vi "Test-Sideways Motors.vi"() -> ()   [LabVIEW 2014, in "Comp Driver.lvlib"]
uses:
  Comp Robot/Comp Drive/Comp Driver.lvlib
  Robot Actor Framework/Trace/Trace Controller Class/Config.ctl
  Comp Robot/Comp Motors with Encoders/Comp Motors with Encoders Class/Motor Controller Config.ctl
  Robot/Motor with Encoders/Motors with Encoders Class/Motors with Encoders Config.ctl
  Comp Robot/Comp Motors with Encoders/Comp Motors with Encoders Class/Encoder Config.ctl
  Comp Robot/Comp Trace Controller/Comp Trace Controller Class/Comp Trace Controller.lvclass
  Comp Robot/Comp Motors with Encoders/Comp Motors with Encoders Class/Comp Motors with Encoders.lvclass
  Comp Robot/Comp Pressure/Comp Pressure Class/Comp Pressure.lvclass
  <vilib>/Rock Robotics/WPI/DriverStation/WPI_DriverStationRobotMode2.ctl
  Robot/Motor with Encoders/Motors with Encoders Messages/Set Rate (Percent) Msg/Set Rate (Percent) Msg.lvclass/Set Rate (Percent) Msg.ctl
  <vilib>/ActorFramework/Message Enqueuer/Message Enqueuer.lvclass/Message Enqueuer.ctl
  <vilib>/ActorFramework/Message Enqueuer/Enqueue.vi
  <vilib>/ActorFramework/Message Priority Queue/Priority Enqueue.vi
  Robot/Motor with Encoders/Motors with Encoders Messages/Set Rate (Percent) Msg/Set Rate (Percent) Msg.lvclass
  <vilib>/ActorFramework/Stop Msg/Stop Msg.lvclass
  <vilib>/ActorFramework/Actor/Actor.lvclass
  Robot Actor Framework/Trace/Trace Controller Class/Trace Controller.lvclass
  Robot/Motor with Encoders/Motors with Encoders Class/Motors with Encoders.lvclass
panel:
  in  "Encoder Config":T1={"P"=1.0, "D"=0.0, "F"=0.01, "I"=0.01, "Reverse Feedback Sensor"=FALSE, "Encoder Codes Per Rev"=256}
  out "Enable Tele":bool caption="Enabled Teleop"
  in  "Stop Test Loop 1":bool=TRUE
  in  "Finish Test":bool=TRUE
  in  "Start Test":bool=TRUE
  in  "Rate (Percent)":dbl(slide)=-1.0 scale=-1.0..1.0
  in  "Motos with Encoder Config":T2={"Counts  Per Revolution"=256, "Invert Encoder Direction"=FALSE, "Diameter of Revolution"=6.0, "Max RPM"=1500.0, "Encoder Control"=TRUE}
  in  "Slave Motor Controller Configs":T3[](array[typedef])=[{"Device Number"=6, "Invert Motor"=FALSE}]
  in  "Master Motor Controller Config":T3={"Device Number"=11, "Invert Motor"=FALSE}
  in  "Trace Controller Config":T4={"Folder Pattern"="/media/sd%s1", "Starting Letter Position"=1, "Min Free Space (MB)"=50.0, "Max Folders to Check"=10, "Trace Level"=enum."Debug"} {"Min Free Space (MB)" format="%#_13g"}
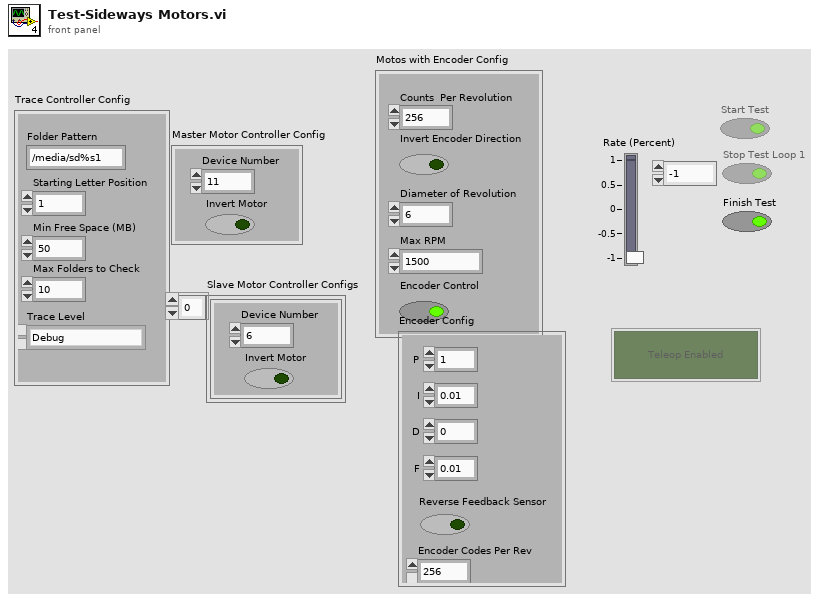
[diagram p1: front panel]
types:
  T1 = typedef "Comp Motors with Encoders.lvlib/Comp Motors with Encoders.lvclass/Encoder Config.ctl" = cluster{"P":dbl, "D":dbl, "F":dbl, "I":dbl, "Reverse Feedback Sensor":bool, "Encoder Codes Per Rev":u16}
  T2 = typedef "Motors with Encoders.lvlib/Motors with Encoders.lvclass/Motors with Encoders Config.ctl" = cluster{"Counts  Per Revolution":u32, "Invert Encoder Direction":bool, "Diameter of Revolution":dbl, "Max RPM":dbl, "Encoder Control":bool}
  T3 = typedef "Comp Motors with Encoders.lvlib/Comp Motors with Encoders.lvclass/Motor Controller Config.ctl" = cluster{"Device Number":u8, "Invert Motor":bool}
  T4 = typedef "Robot Actor Framework.lvlib/Trace.lvlib/Trace Controller.lvclass/Config.ctl" = cluster{"Folder Pattern":string, "Starting Letter Position":i32, "Min Free Space (MB)":dbl, "Max Folders to Check":u32, "Trace Level":enum16{"Critical", "Error", "Warning", "Informational", "Debug"}}
  T5 = enum16{"Critical", "Error", "Warning", "Informational", "Debug"}
  T6 = enum8{"Enabled", "Disabled", "Disabled and Grayed Out"}
  T7 = typedef "WPI_DriverStationRobotMode2.ctl" = enum16{"Autonomous Disabled", "Autonomous Enabled", "Teleop Disabled", "Teleop Enabled", "Disconnected", "Finish", "Test Disabled", "Test Enabled", "Emergency Stopped"}
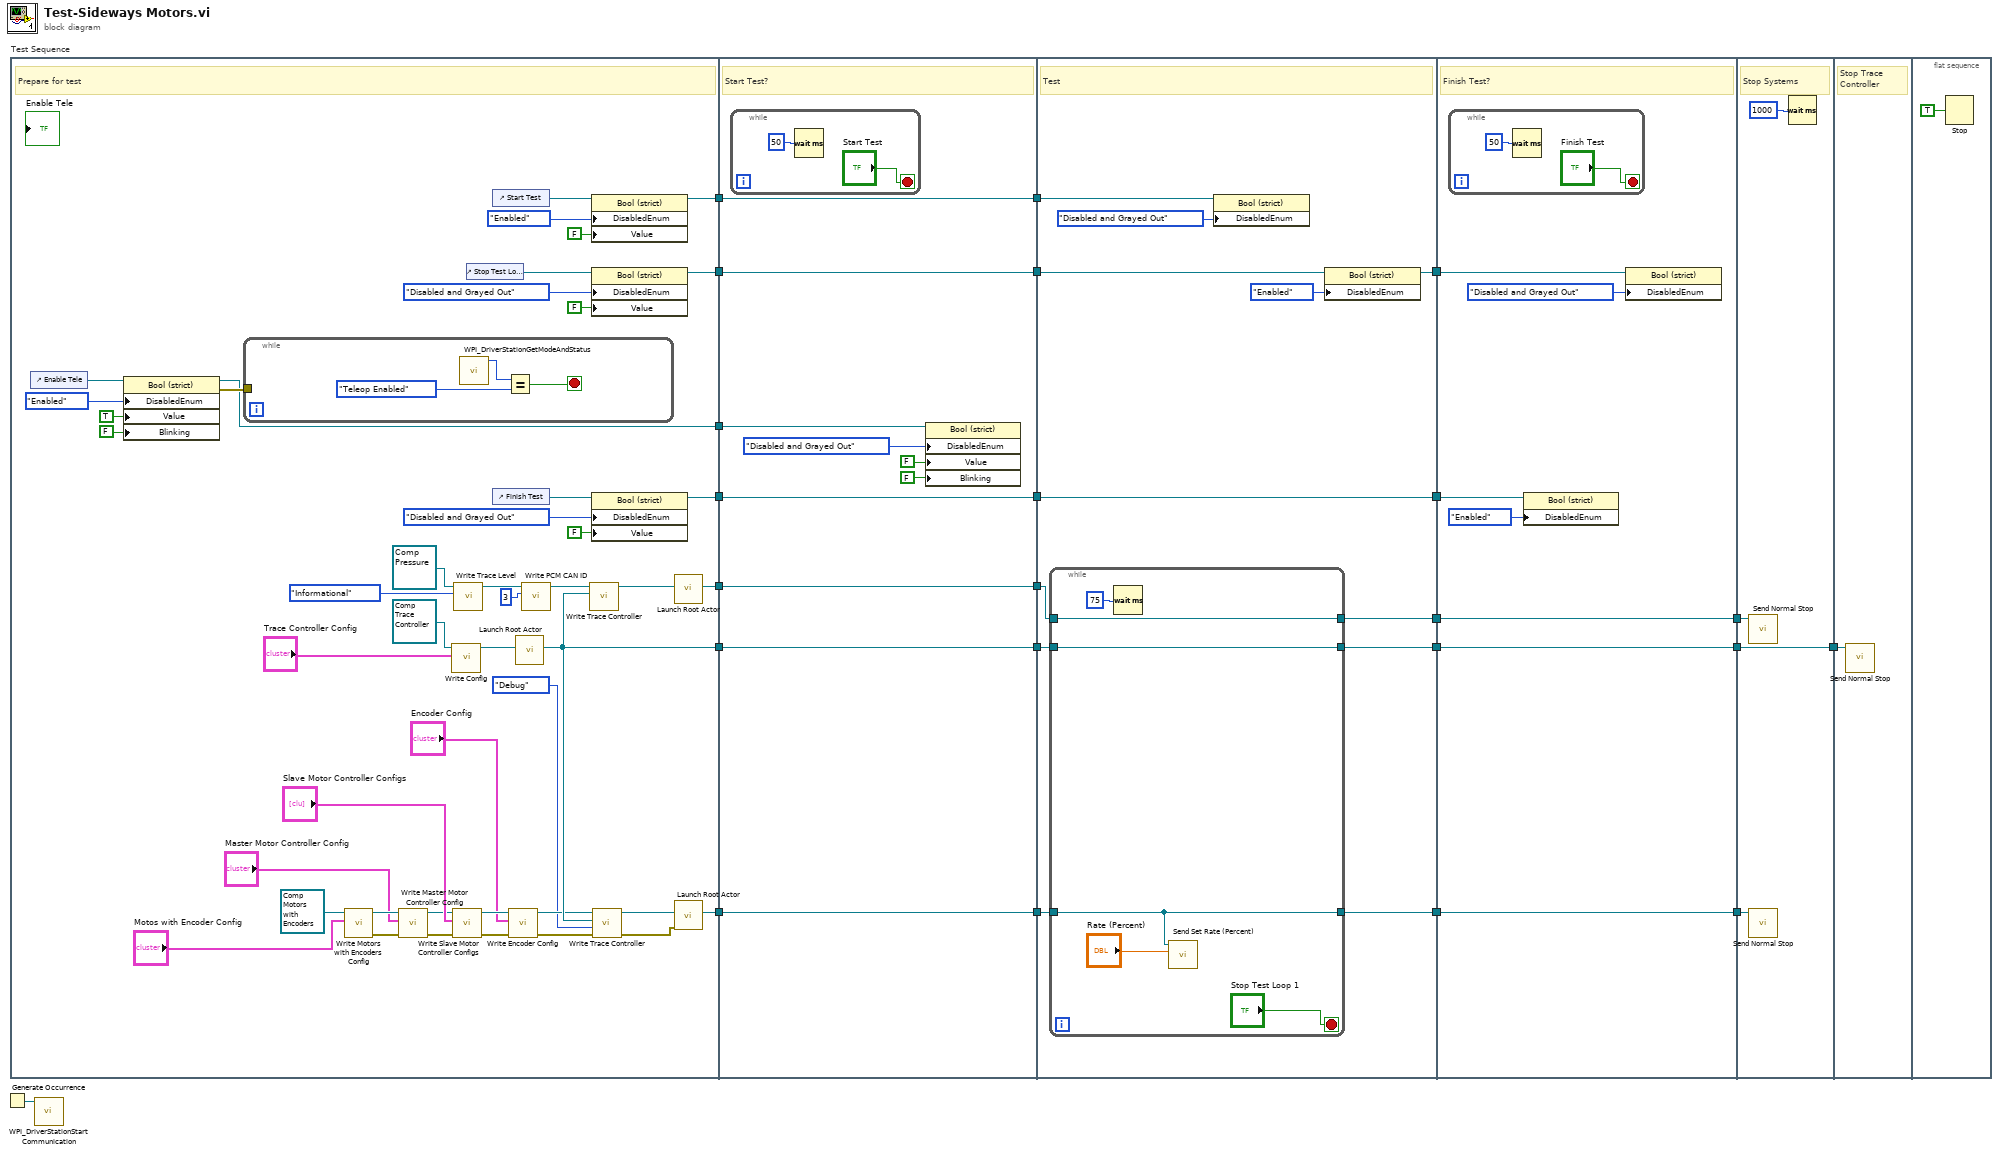
[diagram p0: block diagram]
diagram:
  n1 = Generate Occurrence() -> (w23:refnum<k4>)
  n2 = flat-sequence "Test Sequence" {
    tunnel: [w49] -> w12
    tunnel: [w51] -> w11
    tunnel: [w50] -> w10
    tunnel: [w39] -> w9
    tunnel: [w38] -> w7
    tunnel: [w37] -> w2
    tunnel: [w31] -> w1
    tunnel: [w82] -> w15
    tunnel: [w81] -> w14
    tunnel: [w80] -> w13
    tunnel: w12 -> [w82]
    tunnel: w11 -> [w81]
    tunnel: w10 -> [w80]
    tunnel: w9 -> [w79]
    tunnel: [w79] -> w8
    tunnel: w7 -> [w78]
    tunnel: [w78] -> w6
    tunnel: [w77] -> w3
    tunnel: w2 -> [w77]
    tunnel: w1 -> [w76]
    tunnel: [w91] -> w18
    tunnel: [w93] -> w17
    tunnel: [w92] -> w16
    tunnel: w15 -> [w96]
    tunnel: w14 -> [w94]
    tunnel: w13 -> [w95]
    tunnel: w8 -> [w90]
    tunnel: w6 -> [w88]
    tunnel: [w86] -> w5
    tunnel: [w85] -> w4
    tunnel: w3 -> [w85]
    tunnel: [w109] -> w21
    tunnel: [w108] -> w20
    tunnel: [w107] -> w19
    tunnel: w18 -> [w109]
    tunnel: w17 -> [w108]
    tunnel: w16 -> [w107]
    tunnel: w5 -> [w106]
    tunnel: w4 -> [w103]
    tunnel: [w115] -> w22
    tunnel: w21 -> [w115]
    tunnel: w20 -> [w114]
    tunnel: w19 -> [w112]
    tunnel: w22 -> [w116]
    frame #0 {
      # "Prepare for test"
      n3 = control-ref of="Enable Tele"() -> (w36:refnum<vi>)
      n4 = property class="Bool (strict)"(reference=w36, "DisabledEnum"=T6."Enabled" ("Disabled"), "Value"=TRUE, "Blinking"=FALSE) -> (reference out=w31:refnum<vi>, error out=w33:errorcluster)  [unwired: 1 in]
      n5 = while {
        tunnel: w33 -> [_]
        stop <- w70 stop-if-true
        n6 = call <vilib>:"WPI_DriverStationGetModeAndStatus.vi"() -> ("Robot Mode"=w72:T7)  [unwired: 10 in, 1 out]
        n7 = Equal?(x=w72, y=WPI_DriverStationRobotMode2."Teleop Enabled") -> (x = y?=w70:bool)
      }
      n8 = call-dynamic "Write Motors with Encoders Config.vi"("Motors with Encoders Config"="Motos with Encoder Config", "Motors with Encoders in"=refnum<class "Comp Motors with Encoders.lvclass"> refnum ("Comp Motors with Encoders.lvlib:Comp Motors with Encoders.lvclass")) -> ("error out"=w60:errorcluster, "Motors with Encoders out"=w58:refnum<class "Comp Motors with Encoders.lvclass">)  [unwired: 8 in]
      n9 = call-dynamic "Write Master Motor Controller Config.vi"("error in (no error)"=w60, "Master Motor Controller Config"="Master Motor Controller Config", "Comp Motors with Encoders in"=w58) -> ("error out"=w61:errorcluster, "Comp Motors with Encoders out"=w55:refnum<class "Comp Motors with Encoders.lvclass">)  [unwired: 7 in]
      n10 = call-dynamic "Write Config.vi"("Config"="Trace Controller Config", "Trace Controller in"=refnum<class "Comp Trace Controller.lvclass"> refnum ("Comp Trace Controller.lvlib:Comp Trace Controller.lvclass")) -> ("Trace Controller out"=w54:refnum<class "Comp Trace Controller.lvclass">)  [unwired: 8 in, 1 out]
      n11 = call-dynamic "Write Slave Motor Controller Configs.vi"("error in (no error)"=w61, "Slave Motor Controller Configs"="Slave Motor Controller Configs", "Comp Motors with Encoders in"=w55) -> ("error out"=w28:errorcluster, "Comp Motors with Encoders out"=w30:refnum<class "Comp Motors with Encoders.lvclass">)  [unwired: 7 in]
      n12 = call-dynamic "Write Trace Level.vi"("Trace Level"=T5."Informational", "System Actor in"=refnum<class "Comp Pressure.lvclass"> refnum ("Comp Pressure.lvlib:Comp Pressure.lvclass")) -> ("System Actor out"=w66:refnum<class "Comp Pressure.lvclass">)  [unwired: 8 in, 1 out]
      n13 = control-ref of="Stop Test Loop 1"() -> (w43:refnum<vi>)
      n14 = control-ref of="Start Test"() -> (w48:refnum<vi>)
      n15 = control-ref of="Finish Test"() -> (w42:refnum<vi>)
      n16 = call-dynamic "Write Encoder Config.vi"("error in (no error)"=w28, "Encoder Config"="Encoder Config", "Comp Motors with Encoders in"=w30) -> ("error out"=w27:errorcluster, "Comp Motors with Encoders out"=w29:refnum<class "Comp Motors with Encoders.lvclass">)  [unwired: 7 in]
      n17 = call <vilib>:"Launch Root Actor.vi"("Actor"=w54) -> ("Actor's Enqueuer"=w50:refnum<class "Message Enqueuer.lvclass">)  [unwired: 9 in, 1 out]
      n18 = call-dynamic "Write PCM CAN ID.vi"("PCM CAN ID"=u8 3, "Comp Pressure in"=w66) -> ("Comp Pressure out"=w68:refnum<class "Comp Pressure.lvclass">)  [unwired: 8 in, 1 out]
      n19 = call-dynamic "Write Trace Controller.vi"("Trace Controller"=w50, "System Actor in"=w68) -> ("System Actor out"=w69:refnum<class "Comp Pressure.lvclass">)  [unwired: 8 in, 1 out]
      n20 = property class="Bool (strict)"(reference=w48, "DisabledEnum"=T6."Enabled" ("Disabled"), "Value"=FALSE) -> (reference out=w39:refnum<vi>)  [unwired: 1 in, 1 out]
      n21 = property class="Bool (strict)"(reference=w43, "DisabledEnum"=T6."Disabled and Grayed Out" ("Disabled"), "Value"=FALSE) -> (reference out=w38:refnum<vi>)  [unwired: 1 in, 1 out]
      n22 = property class="Bool (strict)"(reference=w42, "DisabledEnum"=T6."Disabled and Grayed Out" ("Disabled"), "Value"=FALSE) -> (reference out=w37:refnum<vi>)  [unwired: 1 in, 1 out]
      n23 = call-dynamic "Write Trace Controller.vi"("error in (no error)"=w27, "Trace Level"=T5."Debug", "Trace Controller"=w50, "System Actor in"=w29) -> ("error out"=w63:errorcluster, "System Actor out"=w62:refnum<class "Comp Motors with Encoders.lvclass">)  [unwired: 6 in]
      n24 = call <vilib>:"Launch Root Actor.vi"("Actor"=w69) -> ("Actor's Enqueuer"=w51:refnum<class "Message Enqueuer.lvclass">)  [unwired: 9 in, 1 out]
      n25 = call <vilib>:"Launch Root Actor.vi"("error in (no error)"=w63, "Actor"=w62) -> ("Actor's Enqueuer"=w49:refnum<class "Message Enqueuer.lvclass">)  [unwired: 8 in, 1 out]
    }
    frame #1 {
      # "Start Test?"
      n26 = while {
        stop <- "Start Test" stop-if-true
        n27 = Wait (ms)(milliseconds to wait=u32 50) -> ()  [unwired: 1 out]
      }
      n28 = property class="Bool (strict)"(reference=w76, "DisabledEnum"=T6."Disabled and Grayed Out" ("Disabled"), "Value"=FALSE, "Blinking"=FALSE) -> ()  [unwired: 1 in, 2 out]
    }
    frame #2 {
      # "Test"
      n29 = while {
        tunnel: w95 -> [w101]
        tunnel: [w101] -> w91
        tunnel: w96 -> [w97]
        tunnel: [w97] -> w93
        tunnel: w94 -> [w100]
        tunnel: [w100] -> w92
        stop <- "Stop Test Loop 1" stop-if-true
        n30 = Wait (ms)(milliseconds to wait=u32 75) -> ()  [unwired: 1 out]
        n31 = call "Send Set Rate (Percent).vi"("Rate (Percentage)"="Rate (Percent)", "Message Enqueuer"=w97) -> ()  [unwired: 8 in, 2 out]
      }
      n32 = property class="Bool (strict)"(reference=w90, "DisabledEnum"=T6."Disabled and Grayed Out" ("Disabled")) -> ()  [unwired: 1 in, 2 out]
      n33 = property class="Bool (strict)"(reference=w88, "DisabledEnum"=T6."Enabled" ("Disabled")) -> (reference out=w86:refnum<vi>)  [unwired: 1 in, 1 out]
    }
    frame #3 {
      # "Finish Test?"
      n34 = while {
        stop <- "Finish Test" stop-if-true
        n35 = Wait (ms)(milliseconds to wait=u32 50) -> ()  [unwired: 1 out]
      }
      n36 = property class="Bool (strict)"(reference=w103, "DisabledEnum"=T6."Enabled" ("Disabled")) -> ()  [unwired: 1 in, 2 out]
      n37 = property class="Bool (strict)"(reference=w106, "DisabledEnum"=T6."Disabled and Grayed Out" ("Disabled")) -> ()  [unwired: 1 in, 2 out]
    }
    frame #4 {
      # "Stop Systems"
      n38 = call <vilib>:"Send Normal Stop.vi"("Message Enqueuer"=w112) -> ()  [unwired: 10 in, 1 out]
      n39 = call <vilib>:"Send Normal Stop.vi"("Message Enqueuer"=w114) -> ()  [unwired: 10 in, 1 out]
      n40 = Wait (ms)(milliseconds to wait=u32 1000) -> ()  [unwired: 1 out]
    }
    frame #5 {
      # "Stop Trace Controller"
      n41 = call <vilib>:"Send Normal Stop.vi"("Message Enqueuer"=w116) -> ()  [unwired: 10 in, 1 out]
    }
    frame #6 {
      n42 = Stop(stop? (T)=TRUE) -> ()
    }
  }
  n43 = call <vilib>:"WPI_DriverStationStart Communication.vi"("occurrence"=w23) -> ()  [unwired: 1 in, 10 out]
